vi "Write serialNumber.vi"(8 "error in (no error)":errorcluster, 10 "serialNumber":string, 11 "Monochromator in":refnum<class "Monochromator.lvclass">) -> (0 "error out":errorcluster, 3 "Monochromator out":refnum<class "Monochromator.lvclass">)   [LabVIEW 2023, in "Monochromator.lvclass"]
uses:
  Monochromator.lvclass
  Monochromator.lvclass/Monochromator.ctl
  GenericDevice/GenericDevice.lvclass
panel:
  # "Connector Pane"
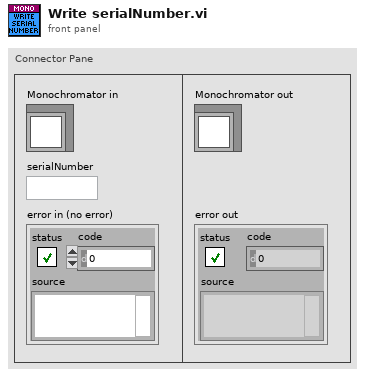
[diagram p1: front panel]
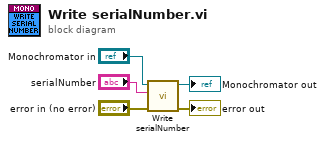
[diagram p0: block diagram]
diagram:
  n1 = call-parent "Write serialNumber.vi"("error in (no error)"="error in (no error)", "serialNumber"="serialNumber", "GenericDevice in"="Monochromator in") -> ("error out"=→"error out":errorcluster, "GenericDevice out"=→"Monochromator out":refnum<class "Monochromator.lvclass">)  [unwired: 7 in]
